vi "ex_openTDMForAppend.vi"(7 "always read cache":bool, 8 "error in (no error)":errorcluster, 9 "Express Wave Attributes Plus in":T1[](array[typedef]) {"dX" format="%.2f"; "X0" format="%<%X\n%x>T"; "Timestamp" format="%<%X\n%x>T"; "Start Timestamp" format="%<%X\n%x>T"}, 10 "file params":T3 {"Flags"."time preference" items=["Absolute", "Relative"]; "Flags"."x_columns" items=["None", "One", "Multiple"]; "origin time" format="%<%X\n%x>T"}, 11 "append info in":T2) -> (0 "error out":errorcluster, 2 "file params out":T3={"delimiter"="\t", "origin time"=timestamp(0 s since 1904-01-01), "Flags"={"include col headings?"=TRUE, "x_columns"=0, "col headings always?"=TRUE, "time preference"=0, "hide col headings"=FALSE}, "Decimal Separator"=""} {"Flags"."time preference" items=["Absolute", "Relative"]; "Flags"."x_columns" items=["None", "One", "Multiple"]; "origin time" format="%<%X\n%x>T"}, 3 "append info out":T2)   [LabVIEW 2020]
uses:
  storage/Storage.llb/__loadPropRefList.vi
  storage/lvStorage.llb/_wf_attributes.ctl
  storage/Storage.llb/__loadPropString.vi
  storage/Storage.llb/__savePropString.vi
  storage/Storage.llb/__loadPropTime.vi
  express/express input/ExFileReadBlock.llb/ex_ReadFileParams.ctl
  express/express output/ExFileWriteBlock.llb/ex_WriteFileParams.ctl
  ex_appendInfoTDM.ctl
  express/express shared/transition.llb/ex_WaveformAttribsPlus.ctl
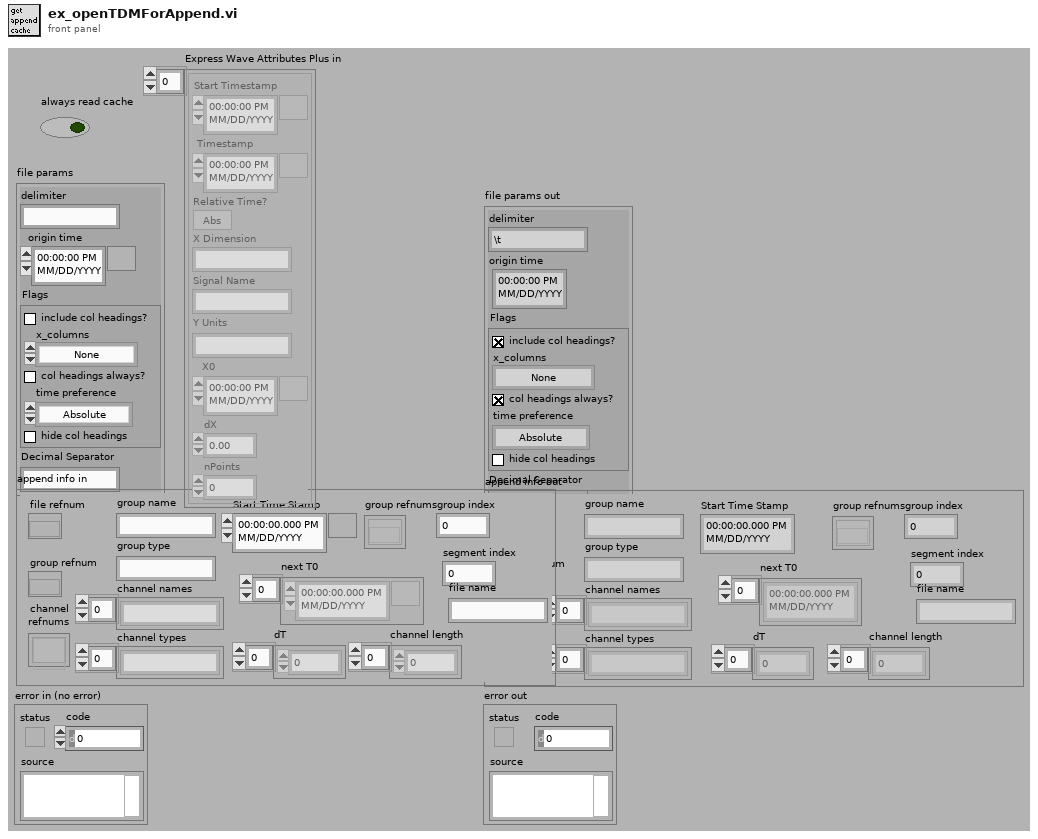
[diagram p1: front panel]
types:
  T1 = typedef "ex_WaveformAttribsPlus.ctl" = cluster{"Start Timestamp":timestamp, "Timestamp":timestamp, "Relative Time?":bool, "X Dimension":string, "Signal Name":string, "Y Units":string, "X0":timestamp, "dX":dbl, "nPoints":i32}
  T2 = typedef "ex_appendInfoTDM.ctl" = cluster{"channel\nrefnums":refnum<k20>[], "channel names":string[], "channel types":string[], "file refnum":refnum<k20>, "group refnum":refnum<k20>, "group name":string, "group type":string, "next T0":timestamp[], "dT":dbl[], "Start Time Stamp":timestamp, "channel length":u32[], "group index":u32, "group refnums":refnum<k20>[], "file name":string, "segment index":u32}
  T3 = typedef "ex_WriteFileParams.ctl" = cluster{"delimiter":string, "origin time":timestamp, "Flags":T4, "Decimal Separator":string}
  T4 = typedef "ex_ReadFileParams.ctl" = cluster{"include col headings?":bool, "x_columns":u16, "col headings always?":bool, "time preference":u16, "hide col headings":bool}
  T5 = typedef "_wf_attributes.ctl" = enum16{"t0", "dt", "X_Name", "X_Unit", "x0", "abs/rel", "nPoints", "file_timestamp", "xcolumns"}
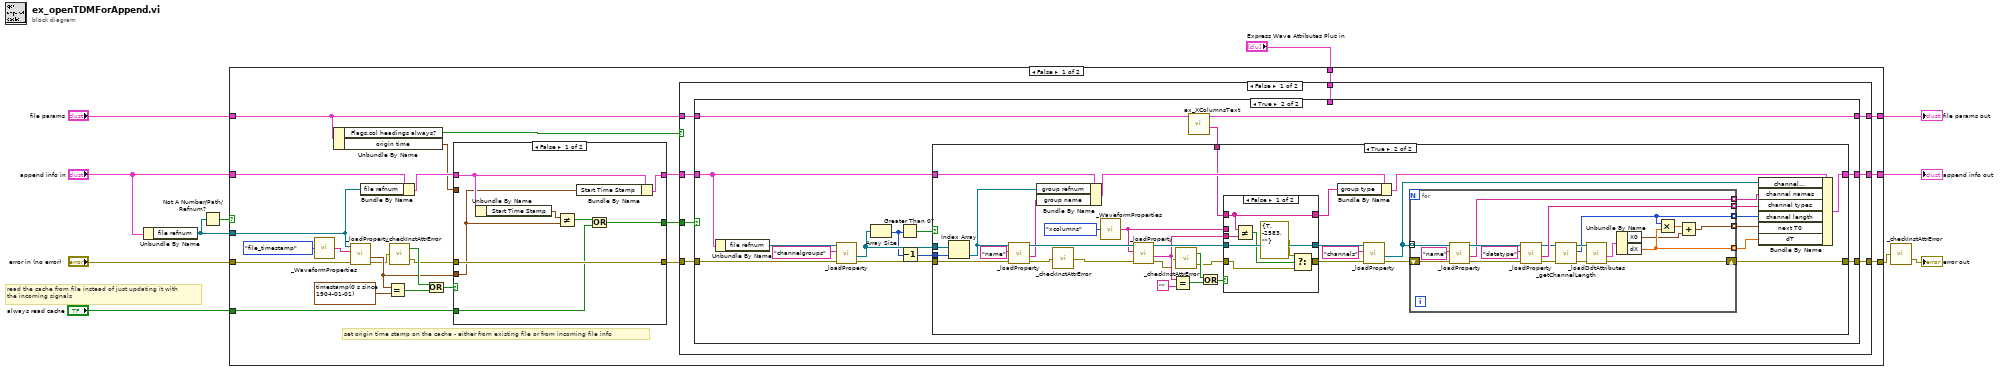
[diagram p0: block diagram]
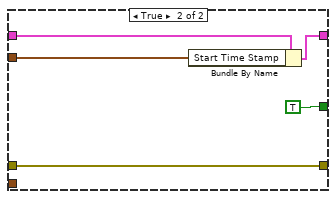
[diagram p2: hidden frame]
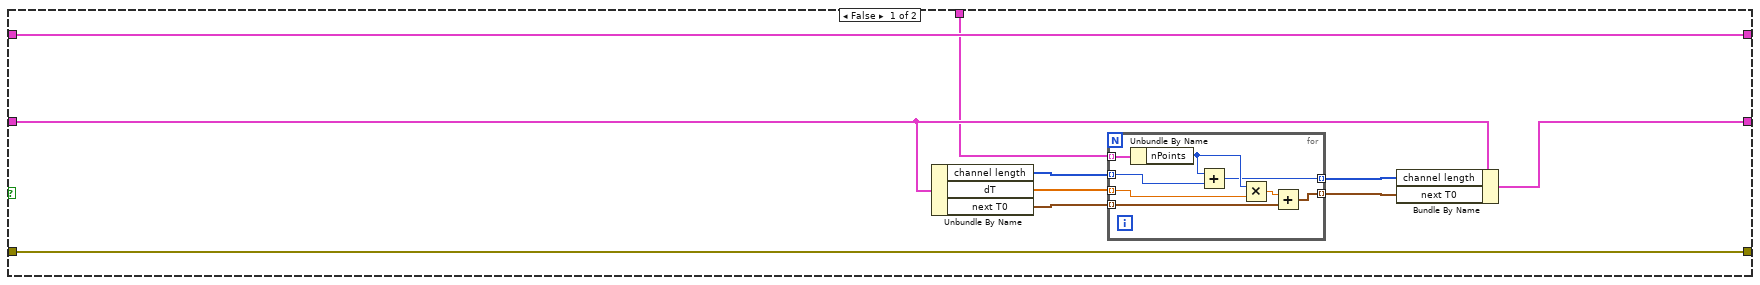
[diagram p3: hidden frame]
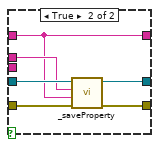
[diagram p5: hidden frame]
diagram:
  # "read the cache from file instead of just updating it with\nthe incoming signals"
  n1 = Unbundle By Name("append info in") -> ("file refnum"=w5:refnum<k20>)
  n2 = Not A Number/Path/Refnum?(number/path/refnum=w5) -> (NaN/Path/Refnum?=w7:bool)
  n3 = case shown="False" w7 {
    tunnel: "error in (no error)" -> [w27 w161]
    tunnel: [w35 w161] -> w2
    tunnel: "file params" -> [w34 w163]
    tunnel: [w32 w163] -> w9
    tunnel: [w31 w162] -> w8
    tunnel: w5 -> [w18 _]
    tunnel: "append info in" -> [w22 w162]
    tunnel: "always read cache" -> [w16 _]
    tunnel: "Express Wave Attributes Plus in" -> [w15 _]
    frame False {
      # "set origin time stamp on the cache - either from existing file or from incoming file info"
      n4 = call "_WaveformProperties.vi"("Property"=_wf_attributes."file_timestamp") -> ("Name"=w30:string)
      n5 = Unbundle By Name(w34) -> ("Flags.col headings always?"=w33:bool, "origin time"=w20:timestamp)
      n6 = call-poly "_loadProperty.vi"("error in (no error)"=w27, "Property name"=w30, "storage refnum"=w18) -> ("error out"=w13:errorcluster, "Value"=w23:timestamp)  [unwired: 7 out]
      n7 = Bundle By Name(cluster=w22, "file refnum"=w18) -> (w21:T2)
      n8 = Equal?(x=w23, y=timestamp(0 s since 1904-01-01)) -> (x = y?=w25:bool)
      n9 = call "_checkInstAttrError.vi"("error in (no error)"=w13) -> ("Create?"=w24:bool, "error out"=w14:errorcluster)
      n10 = Or(x=w24, y=w25) -> (x .or. y?=w28:bool)
      n11 = case shown="False" w28 {
        tunnel: [w43 w48] -> w12
        tunnel: w14 -> [w43 w48]
        tunnel: w23 -> [w39 _]
        tunnel: w21 -> [w40 w45]
        tunnel: w20 -> [_ w47]
        tunnel: [w42 w46] -> w19
        tunnel: [w37 TRUE] -> w17
        tunnel: w16 -> [w36 _]
        frame False {
          n12 = Unbundle By Name(w40) -> ("Start Time Stamp"=w41:timestamp)
          n13 = Not Equal?(x=w41, y=w39) -> (x != y?=w38:bool)
          n14 = Bundle By Name(cluster=w40, "Start Time Stamp"=w39) -> (w42:T2)
          n15 = Or(x=w38, y=w36) -> (x .or. y?=w37:bool)
        }
        frame True {
          n16 = Bundle By Name(cluster=w45, "Start Time Stamp"=w47) -> (w46:T2)
        }
      }
      n17 = case shown="False" w33 {
        tunnel: [w56 w158] -> w31
        tunnel: w34 -> [w52 w160]
        tunnel: [w55 w159] -> w35
        tunnel: [w51 w160] -> w32
        tunnel: w12 -> [w54 w159]
        tunnel: w19 -> [w53 w158]
        tunnel: w17 -> [w50 _]
        tunnel: w15 -> [w49 _]
        frame False {
          n18 = case shown="True" w50 {
            tunnel: [w64 w88] -> w56
            tunnel: [w59 w87] -> w55
            tunnel: w54 -> [w59 w80]
            tunnel: w53 -> [w62 w78]
            tunnel: w52 -> [w63 w77]
            tunnel: [w63 w76] -> w51
            tunnel: w49 -> [w57 _]
            frame False {
              n19 = Unbundle By Name(w62) -> ("channel length"=w61:u32[], "dT"=w60:dbl[], "next T0"=w58:timestamp[])
              n20 = for {
                tunnel: [w68] -> w66 mode=indexing
                tunnel: [w73] -> w65 mode=indexing
                tunnel: w61 -> [w69] mode=indexing
                tunnel: w60 -> [w72] mode=indexing
                tunnel: w57 -> [w71] mode=indexing
                tunnel: w58 -> [w67] mode=indexing
                n21 = Unbundle By Name(w71) -> ("nPoints"=w70:i32)
                n22 = Add(x=w70, y=w69) -> (x+y=w68:u32)
                n23 = Multiply(x=w70, y=w72) -> (x*y=w74:dbl)
                n24 = Add(x=w74, y=w67) -> (x+y=w73:timestamp)
              }
              n25 = Bundle By Name(cluster=w62, "channel length"=w66, "next T0"=w65) -> (w64:T2)
            }
            frame True {
              n26 = Unbundle By Name(w78) -> ("file refnum"=w79:refnum<k20>)
              n27 = call-poly "_loadProperty.vi"("error in (no error)"=w80, "Property name"="channelgroups", "storage refnum"=w79) -> ("error out"=w81:errorcluster, "Value"=w85:refnum<k20>[])  [unwired: 7 out]
              n28 = Array Size(array=w85) -> (size(s)=w82:i32)
              n29 = Greater Than 0?(x=w82) -> (x > 0?=w84:bool)
              n30 = Decrement(x=w82) -> (x-1=w83:i32)
              n31 = call "ex_XColumnsText.vi"("file info in"=w77) -> ("xcolumns"=w75:string, "file info out"=w76:T3)  [unwired: 5 out]
              n32 = case shown="True" w84 {
                tunnel: w85 -> [_ w125]
                tunnel: w83 -> [_ w124]
                tunnel: w81 -> [w90 w121]
                tunnel: [w90 w102] -> w87
                tunnel: [w89 w100] -> w88
                tunnel: w78 -> [w89 w113]
                tunnel: w75 -> [_ w107]
                frame False {
                }
                frame True {
                  n33 = Index Array(array=w125, index=w124) -> (element=w104:refnum<k20>)
                  n34 = call-poly "_loadProperty.vi"("error in (no error)"=w121, "Property name"="name", "storage refnum"=w104) -> ("error out"=w93:errorcluster, "Value"=w115:string, "dup storage refnum"=w120:refnum<k20>)  [unwired: 6 out]
                  n35 = Bundle By Name(cluster=w113, "group refnum"=w104, "group name"=w115) -> (w114:T2)
                  n36 = call "_checkInstAttrError.vi"("error in (no error)"=w93) -> ()  [unwired: 2 out]
                  n37 = call "_WaveformProperties.vi"("Property"=_wf_attributes."xcolumns") -> ("Name"=w110:string)
                  n38 = call-poly "_loadProperty.vi"("error in (no error)"=w93, "Property name"=w110, "storage refnum"=w120) -> ("error out"=w92:errorcluster, "Value"=w108:string, "dup storage refnum"=w111:refnum<k20>)  [unwired: 6 out]
                  n39 = Equal?(x=w108, y="") -> (x = y?=w116:bool)
                  n40 = call "_checkInstAttrError.vi"("error in (no error)"=w92) -> ("Create?"=w117:bool, "error out"=w91:errorcluster)
                  n41 = Or(x=w117, y=w116) -> (x .or. y?=w112:bool)
                  n42 = case shown="False" w112 {
                    tunnel: w91 -> [w147 w157]
                    tunnel: w111 -> [w151 w156]
                    tunnel: w110 -> [_ w155]
                    tunnel: [w149 w152] -> w109
                    tunnel: [w146 w154] -> w106
                    tunnel: [w151 w153] -> w105
                    tunnel: w108 -> [w150 _]
                    tunnel: w107 -> [w149 w152]
                    frame False {
                      n43 = Not Equal?(x=w149, y=w150) -> (x != y?=w148:bool)
                      n44 = Select(t=errorcluster {"status"=TRUE, "code"=-2583, "source"=""} ("error out"), s=w148, f=w147) -> (s? t:f=w146:errorcluster)
                    }
                    frame True {
                      n45 = call-poly "_saveProperty.vi"("error in (no error)"=w157, "Value"=w152, "Property name"=w155, "storage refnum"=w156) -> ("error out"=w154:errorcluster, "dup storage refnum"=w153:refnum<k20>)  [unwired: 1 in, 5 out]
                    }
                  }
                  n46 = Bundle By Name(cluster=w114, "group type"=w109) -> (w101:T2)
                  n47 = call-poly "_loadProperty.vi"("error in (no error)"=w106, "Property name"="channels", "storage refnum"=w105) -> ("error out"=w103:errorcluster, "Value"=w99:refnum<k20>[])  [unwired: 7 out]
                  n48 = for {
                    tunnel: w99 -> [w143] mode=indexing
                    shift-right: [w133] -> w102
                    shift-left: w103 -> [w144]
                    tunnel: [w138] -> w98 mode=indexing
                    tunnel: [w137] -> w97 mode=indexing
                    tunnel: [w130] -> w96 mode=indexing
                    tunnel: [w129] -> w95 mode=indexing
                    tunnel: [w126] -> w94 mode=indexing
                    n49 = call-poly "_loadProperty.vi"("error in (no error)"=w144, "Property name"="name", "storage refnum"=w143) -> ("error out"=w141:errorcluster, "Value"=w138:string, "dup storage refnum"=w139:refnum<k20>)  [unwired: 6 out]
                    n50 = call-poly "_loadProperty.vi"("error in (no error)"=w141, "Property name"="datatype", "storage refnum"=w139) -> ("error out"=w135:errorcluster, "Value"=w137:string, "dup storage refnum"=w136:refnum<k20>)  [unwired: 6 out]
                    n51 = call "_getChannelLength.vi"("error in (no error)"=w135, "channel refnum in"=w136) -> ("error out"=w134:errorcluster, "channel length"=w130:i32, "channel refnum out"=w132:refnum<k20>)  [unwired: 3 out]
                    n52 = call "_loadDdtAttributes.vi"("error in (no error)"=w134, "Channel in"=w132) -> ("error out"=w133:errorcluster, "output cluster"=w131:T1)  [unwired: 4 out]
                    n53 = Unbundle By Name(w131) -> ("X0"=w127:timestamp, "dX"=w129:dbl)
                    n54 = Multiply(x=w130, y=w129) -> (x*y=w128:dbl)
                    n55 = Add(x=w128, y=w127) -> (x+y=w126:timestamp)
                  }
                  n56 = Bundle By Name(cluster=w101, "channel\nrefnums"=w99, "channel names"=w98, "channel types"=w97, "channel length"=w96, "next T0"=w94, "dT"=w95) -> (w100:T2)
                }
              }
            }
          }
        }
        frame True {
        }
      }
    }
    frame True {
    }
  }
  "file params out" <- w9
  "append info out" <- w8
  n57 = call "_checkInstAttrError.vi"("error in (no error)"=w2) -> ("error out"=→"error out":errorcluster)  [unwired: 1 out]
